vi "Ramp Pattern.vi"   [LabVIEW 2014, in "NI_AALBase.lvlib"]
doc: "Generates an array containing a ramp pattern. You must manually select the polymorphic instance you want to use."
uses:
  NI_AALBase.lvlib
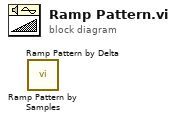
[diagram p0: block diagram]
diagram:
  n1 = call "Ramp Pattern by Samples.vi"() -> ()  [unwired: 10 in, 2 out]
  n2 = call "Ramp Pattern by Delta.vi"() -> ()  [unwired: 9 in, 3 out]
